vi "Matrix Subtract and show result.vi"() -> ()   [LabVIEW 2014, in "Arduino MatrixMath.lvlib"]
uses:
  <vilib>/Aledyne-TSXperts/Arduino Compatible Compiler for LabVIEW/addons/Arduino MatrixMath/Arduino MatrixMath.lvlib
  <vilib>/Aledyne-TSXperts/Arduino Compatible Compiler for LabVIEW/Arduino Compatible Compiler for LabVIEW.lvlib
panel:
  in  "A":sgl[](array[numeric])=[1.0, 2.0, 3.0, 4.0, 5.0, 6.0, 7.0, 8.0]
  in  "B":sgl[](array[numeric])=[1.0, 2.0, 3.0, 4.0, 5.0, 6.0, 7.0, 8.0]
  out "Error Out":errorcluster
  in  "Error In":errorcluster
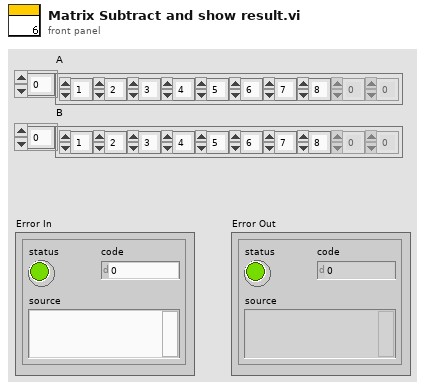
[diagram p1: front panel]
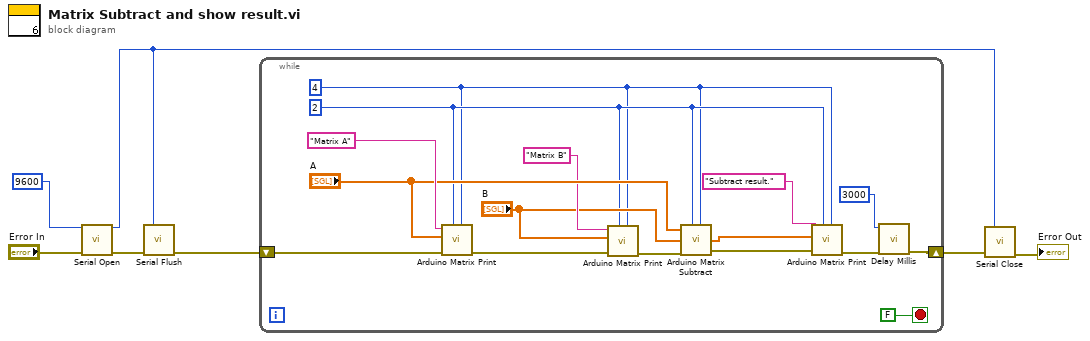
[diagram p0: block diagram]
diagram:
  n1 = call <vilib>:"Serial Open.vi"("Speed"=u32 9600, "error in (no error)"="Error In") -> ("Instance"=w1:u8, "error out"=w3:errorcluster)  [unwired: 12 in]
  n2 = call <vilib>:"Serial Flush.vi"("Instance"=w1, "error in (no error)"=w3) -> ("error out"=w2:errorcluster)  [unwired: 13 in]
  n3 = while {
    shift-right: [w19] -> w7
    shift-left: w2 -> [w22]
    stop <- FALSE stop-if-true
    w8 = u8 4 ("cols num.")
    w9 = u8 2 ("rows num.")
    n4 = call <vilib>:"Arduino Matrix Print.vi"("cols num."=w8, "rows num."=w9, "Error In"=w22, "A"="A", "Label"="Matrix A") -> ("Error Out"=w13:errorcluster)  [unwired: 6 in]
    n5 = call <vilib>:"Arduino Matrix Print.vi"("cols num."=w8, "rows num."=w9, "Error In"=w13, "A"="B", "Label"="Matrix B") -> ("Error Out"=w12:errorcluster)  [unwired: 6 in]
    n6 = call <vilib>:"Arduino Matrix Subtract.vi"("A"="A", "rows num."=w9, "B"="B", "Error In"=w12, "cols num."=w8) -> ("A-B"=w14:sgl[], "Error Out"=w16:errorcluster)  [unwired: 3 in]
    n7 = call <vilib>:"Arduino Matrix Print.vi"("cols num."=w8, "rows num."=w9, "Error In"=w16, "A"=w14, "Label"="Subtract result.") -> ("Error Out"=w18:errorcluster)  [unwired: 6 in]
    n8 = call <vilib>:"Delay Millis.vi"("error in (no error)"=w18, "delay"=u32 3000) -> ("error out"=w19:errorcluster)  [unwired: 9 in]
  }
  n9 = call <vilib>:"Serial Close.vi"("Instance"=w1, "error in (no error)"=w7) -> ("error out"=→"Error Out":errorcluster)  [unwired: 13 in]
